vi "ADIS16448_RoboRIO_Teensy_Open.vi"(7 "error in":errorcluster) -> (0 "error out":errorcluster, 3 "SerialPortRef":T1)   [LabVIEW 2015, in "RoboRIO-Teensy-ADIS16448-Interface.lvlib"]
uses:
  RoboRIO-Teensy-ADIS16448-Interface.lvlib
  <vilib>/Rock Robotics/WPI/SerialPort/WPI_SerialPortRef.ctl
  <vilib>/Rock Robotics/WPI/SerialPort/WPI_SerialPort.ctl
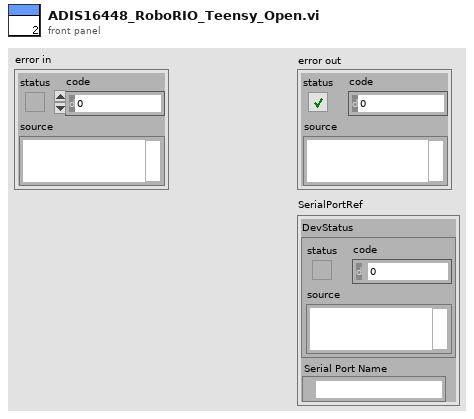
[diagram p1: front panel]
types:
  T1 = typedef "WPI_SerialPortRef.ctl" = cluster{"DevStatus":errorcluster, "Serial Port Name":refnum<visa-resource-name>}
  T2 = typedef "WPI_SerialPort.ctl" = enum16{"Onboard RS-232", "MXP TTL"}
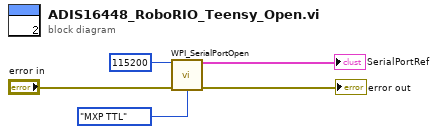
[diagram p0: block diagram]
diagram:
  n1 = call <vilib>:"WPI_SerialPortOpen.vi"("Baud Rate"=u32 115200, "error in (no error)"="error in", "Serial Port"=WPI_SerialPort."MXP TTL") -> ("SerialPortRef"=→"SerialPortRef":T1, "error out"=→"error out":errorcluster)  [unwired: 11 in]
